vi "FileNameGenerator.vi"(5 "Type of scan":T1, 6 "Case temp":string, 7 "Add Axis":bool, 8 "Current Plane in":i32, 9 "String in":refnum<vi>, 10 "Boolean":bool, 11 "Case Name in":string) -> (0 "Current Plane out":i32, 2 "Root Case Name":string, 3 "Case Name out":string)   [LabVIEW 2022 SP3]
uses:
  ScanningControl/-ScanSystem/Controls/ScanType2.ctl
  ScanningControl/Motion Controllers/-MotionRoutines/MotionGlobals.vi
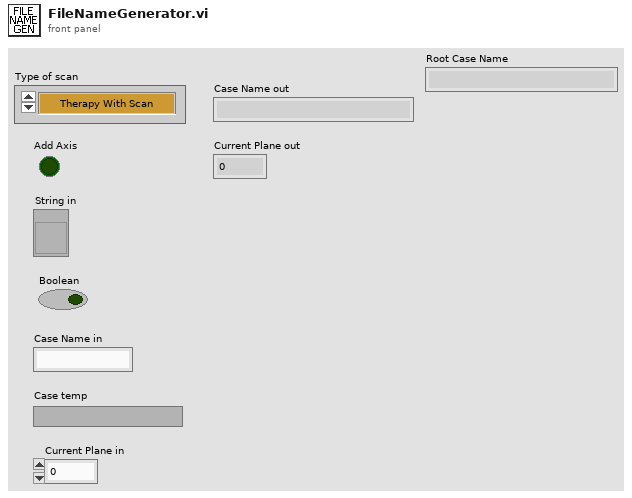
[diagram p1: front panel]
types:
  T1 = typedef "ScanType2.ctl" = enum16{"Therapy With Scan", "M scan", "M Scan With Therapy Burst", "1-D B Scan", "1-D B Scan With Therapy Burst", "2-D B Scan", "2-D B Scan With Therapy Burst", "Rotational Scan", "1-D B-Scan PRF", "2-D B-Scan PRF", "Real-Time Scan", "Contrast Agents", "1-D w/ Real-Time Set Up", "Dual Transducer", "Acoustic Microscopy", "Hydrophone Scanning"}
  T2 = typedef "location.ctl" = enum16{"Automatic", "WCM Main", "Hawaii", "Columbia MM3000", "Columbia  NI System", "NYU", "RRI 2", "UHI Allen", "CUMC RT", "Chiba", "Stony Brook", "WCM Microscopy", "WCM Aeoretch", "WCM Optics Lab", "WCM Main 2Axis", "WCM Rotation", "WCM SAM SMAC", "SERI GP"}
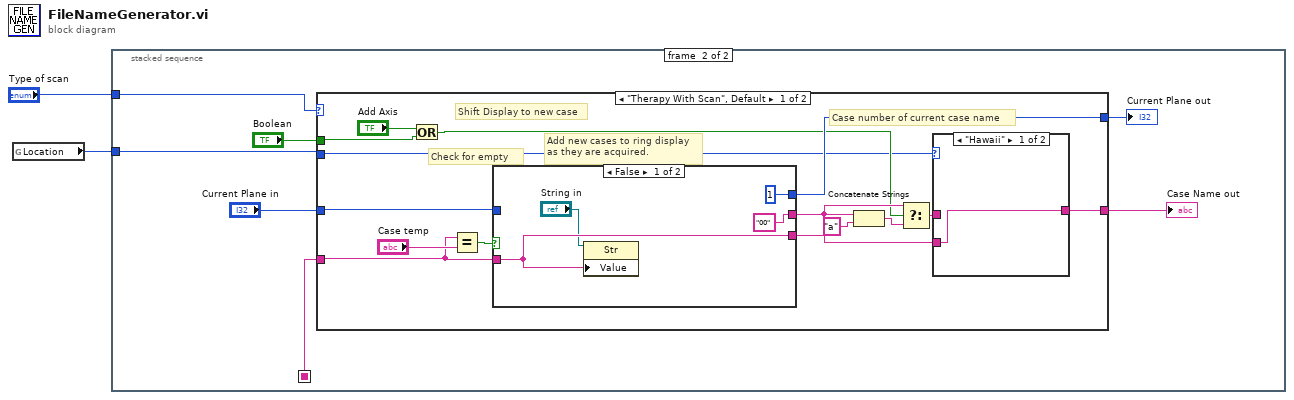
[diagram p0: block diagram]
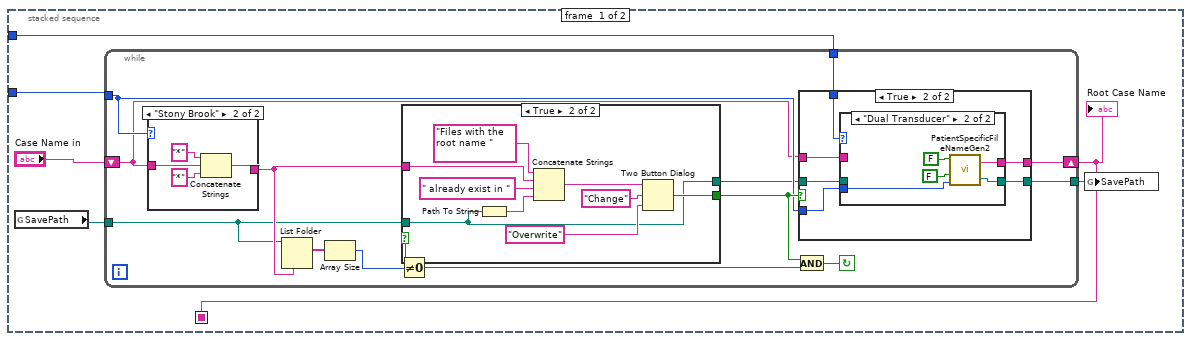
[diagram p2: hidden frame]
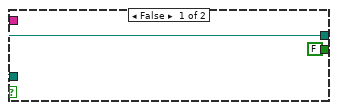
[diagram p3: hidden frame]
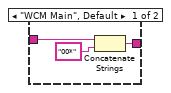
[diagram p4: hidden frame]
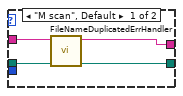
[diagram p6: hidden frame]
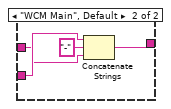
[diagram p7: hidden frame]
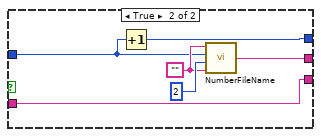
[diagram p8: hidden frame]
diagram:
  n1 = global read "MotionGlobals.vi" "Location"() -> (w2:T2)
  n2 = stacked-sequence {
    seq-local: [w5 _] -> [_ w59]
    tunnel: w2 -> [w4 w58]
    tunnel: "Type of scan" -> [w3 w57]
    frame #0 {
      n3 = global read "MotionGlobals.vi" "SavePath"() -> (w7:path)
      n4 = while {
        shift-right: [w21] -> w5
        shift-left: "Case Name in" -> [w10]
        tunnel: w4 -> [w17]
        tunnel: w7 -> [w13]
        tunnel: [w12] -> w6
        tunnel: w3 -> [w9]
        stop <- w19 continue-if-true
        n5 = case shown="\"Stony Brook\"" w17 {
          tunnel: [w33 w37] -> w16
          tunnel: w10 -> [w34 w36]
          frame "WCM Main", Default {
            n6 = Concatenate Strings(w34, "00*") -> (w33:string)
          }
          frame "Stony Brook" {
            n7 = Concatenate Strings("*" ("string"), w36, "*" ("string")) -> (w37:string)
          }
        }
        n8 = List Folder(path=w13, pattern=w16) -> (filenames=w15:string[])  [unwired: 1 in, 4 out]
        n9 = Array Size(array=w15) -> (size(s)=w14:i32)
        n10 = Not Equal To 0?(x=w14) -> (x != 0?=w20:bool)
        n11 = case shown="True" w20 {
          tunnel: [FALSE ("T button?") w29] -> w18
          tunnel: w13 -> [w22 w24]
          tunnel: w16 -> [_ w27]
          tunnel: [w22 w24] -> w11
          frame False {
          }
          frame True {
            n12 = Path To String(path=w24) -> (string=w25:string)
            n13 = Concatenate Strings("Files with the root name ", w27, " already exist in ", w25) -> (w28:string)
            n14 = Two Button Dialog(message=w28, 1:"Overwrite" ("F button name (\"Cancel\")"), 2:"Change" ("T button name (\"OK\")")) -> (T button?=w29:bool)
          }
        }
        n15 = And(x=w18, y=w20) -> (x .and. y?=w19:bool)
        n16 = case shown="True" w18 {
          tunnel: [w41 w47] -> w21
          tunnel: w10 -> [w41 w46]
          tunnel: w17 -> [_ w43]
          tunnel: [w40 w44] -> w12
          tunnel: w11 -> [w40 w45]
          tunnel: w9 -> [_ w42]
          frame False {
          }
          frame True {
            n17 = case shown="\"Dual Transducer\"" w42 {
              tunnel: [w51 w54] -> w47
              tunnel: w46 -> [w50 _]
              tunnel: w45 -> [w49 _]
              tunnel: [w48 w53] -> w44
              tunnel: w43 -> [_ w52]
              frame "M scan", Default {
                n18 = call "FileNameDuplicatedErrHandler.vi"("Save Path (use dialog)"=w49, "File Name"=w50) -> ("Save Path Out"=w48:path, "File Name Out"=w51:string)  [unwired: 8 in]
              }
              frame "Dual Transducer" {
                n19 = call "PatientSpecificFileNameGen2.vi"("Location"=w52, "Add to Database"=FALSE, "Auto Increment"=FALSE) -> ("SavePathOut"=w53:path, "PatientFileName"=w54:string)  [unwired: 1 in]
              }
            }
          }
        }
      }
      "Root Case Name" <- w5
      n20 = global write "MotionGlobals.vi" "SavePath"(w6) -> ()
    }
    frame #1 {
      n21 = case shown="\"Therapy With Scan\", Default" w57 {
        tunnel: "Boolean" -> [w67 _]
        tunnel: "Current Plane in" -> [w73 w95]
        tunnel: [w72 w95] -> w61
        tunnel: [w71 w94] -> w60
        tunnel: w59 -> [w69 w94]
        tunnel: w58 -> [w64 _]
        frame "Therapy With Scan", Default {
          # "Check for empty"
          # "Case number of current case name"
          # "Shift Display to new case"
          # "Add new cases to ring display\nas they are acquired."
          n22 = Or(x="Add Axis", y=w67) -> (x .or. y?=w68:bool)
          n23 = Equal?(x=w69, y="Case temp") -> (x = y?=w77:bool)
          n24 = case shown="False" w77 {
            tunnel: w73 -> [_ w88]
            tunnel: [1 w89] -> w72
            tunnel: w69 -> [w87 w93]
            tunnel: [w87 w93] -> w76
            tunnel: ["00" ("Numbered File") w91] -> w70
            frame False {
              n25 = property class="Str"(reference="String in", "Value"=w87) -> ()  [unwired: 1 in, 2 out]
            }
            frame True {
              w90 = ""
              n26 = Increment(x=w88) -> (x+1=w89:i32)
              n27 = call "NumberFileName.vi"("String"=w90, "Digits"=2, "File number"=w88, "file name"=w90) -> ("Numbered File"=w91:string)
            }
          }
          n28 = Concatenate Strings(w70, "a") -> (w74:string)
          n29 = Select(t=w70, s=w68, f=w74) -> (s? t:f=w65:string)
          n30 = case shown="\"Hawaii\"" w64 {
            tunnel: w76 -> [w79 w83]
            tunnel: [w79 w82] -> w71
            tunnel: w65 -> [_ w81]
            frame "Hawaii" {
            }
            frame "WCM Main", Default {
              n31 = Concatenate Strings(w83, "-" ("string"), w81) -> (w82:string)
            }
          }
        }
        frame "Real-Time Scan" {
          # "Leave file numbering alone for real-time mode."
        }
      }
      "Case Name out" <- w60
      "Current Plane out" <- w61
    }
  }
